vi "BandwidthСalc (SubVI).vi"(10 "Freq":dbl, 11 "NTick":i32) -> (1 "norm":bool, 2 "Mbit/s":string, 3 "T_sum":dbl)   [LabVIEW 2017]
panel:
  in  "y":dbl=0.00085 format="%#_13g"
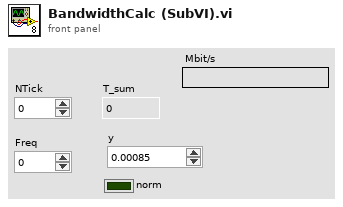
[diagram p1: front panel]
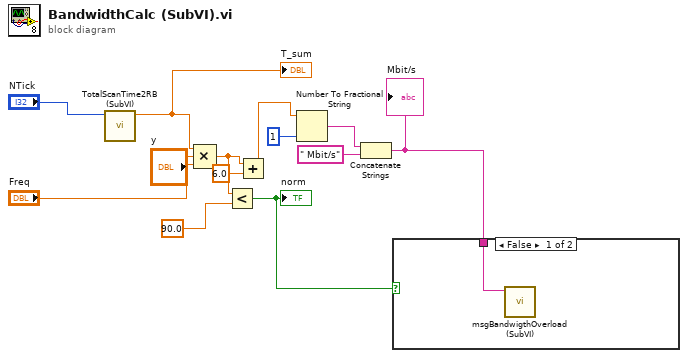
[diagram p0: block diagram]
diagram:
  n1 = call "TotalScanTime2RB (SubVI).vi"("NTick"="NTick") -> ("T_sum"=w11:dbl)  [unwired: 10 in]
  "T_sum" <- w11
  n2 = Compound Arithmetic op=MULTIPLY(w11, "y", "Freq") -> (w3:dbl)
  n3 = Less?(x=w3, y=90.0) -> (x < y?=w5:bool)
  "norm" <- w5
  n4 = Add(x=w3, y=6.0) -> (x+y=w1:dbl)
  n5 = Number To Fractional String(number=w1, precision (6)=i16 1) -> (F-format string=w7:string)  [unwired: 2 in]
  n6 = Concatenate Strings(w7, " Mbit/s" ("string")) -> (w4:string)
  "Mbit/s" <- w4
  n7 = case shown="False" w5 {
    tunnel: w4 -> [w14 _]
    frame False {
      n8 = call "msgBandwigthOverload (SubVI).vi"("Mbit/s"=w14) -> ()  [unwired: 11 in]
    }
    frame True {
    }
  }
